vi "Get Away Status.vi"(7 "Use Cached Data?":bool, 8 "Error In":errorcluster, 10 "Structure Name":string, 11 "Nest Config":T1) -> (0 "Error Out":errorcluster, 2 "Away?":bool, 3 "Nest Config":T1)   [LabVIEW 2013, in "LMH-Nest.lvlib"]
doc: "Get the status of the specified structure (home or away)."
uses:
  LMH-Nest.lvlib
  Private/Type Defs/Nest Config.ctl
  <vilib>/httpClient/ClientHandle.ctl
  Private/Type Defs/Session Data.ctl
  <vilib>/httpClient/LabVIEWHTTPClient.lvlib
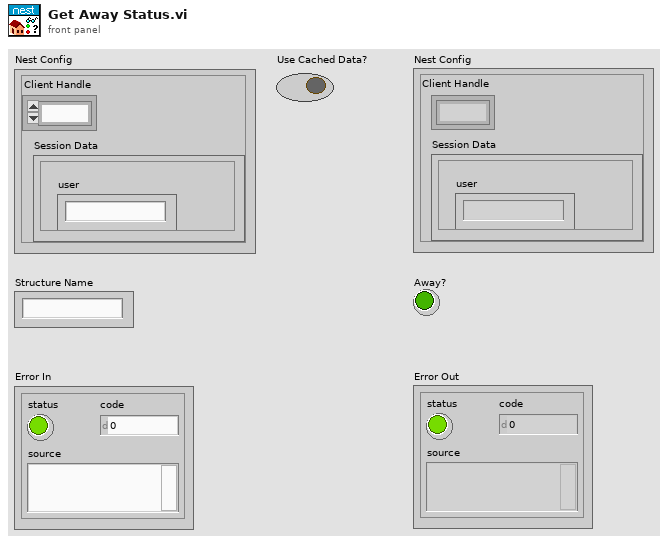
[diagram p1: front panel]
types:
  T1 = typedef "LMH-Nest.lvlib/Nest Config.ctl" = cluster{"Client Handle":T2, "Session Data":T3}
  T2 = typedef "LabVIEWHTTPClient.lvlib/ClientHandle.ctl" = refnum<k1>
  T3 = typedef "LMH-Nest.lvlib/Session Data.ctl" = cluster{"is_superuser":bool, "is_staff":bool, "urls":cluster{"transport_url":string, "rubyapi_url":string, "weather_url":string, "log_upload_url":string, "support_url":string}, "limits":cluster{"thermostats_per_structure":u32, "structures":u32, "thermostats":u32, "smoke_detectors":u32, "smoke_detectors_per_structure":u32}, "access_token":string, "userid":string, "expires_in":string, "email":string, "user":string, "language":string}
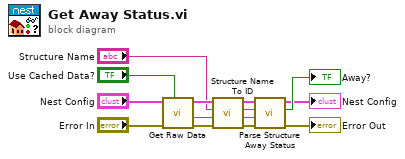
[diagram p0: block diagram]
diagram:
  n1 = call "Get Raw Data.vi"("Use Cached Data?"="Use Cached Data?", "Error In"="Error In", "Nest Config"="Nest Config") -> ("Error Out"=w8:errorcluster, "Data"=w14:string, "Nest Config"=w13:T1)  [unwired: 6 in]
  n2 = call "Structure Name To ID.vi"("Error In"=w8, "Data"=w14, "Structure Name"="Structure Name", "Nest Config"=w13) -> ("Error Out"=w12:errorcluster, "Data"=w11:string, "Structure ID"=w10:string, "Nest Config"=w9:T1)  [unwired: 4 in]
  n3 = call "Parse Structure Away Status.vi"("Error In"=w12, "Data"=w11, "Structure ID"=w10, "Nest Config"=w9) -> ("Error Out"=→"Error Out":errorcluster, "Away?"=→"Away?":bool, "Nest Config"=→"Nest Config":T1)  [unwired: 4 in, 1 out]
